vi "Math-Simple Histogram.vi"(0 "Array":dbl[](array[numeric]), 5 "Binwidth":dbl) -> (4 "Histogram Graph":T1)   [LabVIEW 2020]
uses:
  <vilib>/Analysis/NI_AALPro.lvlib
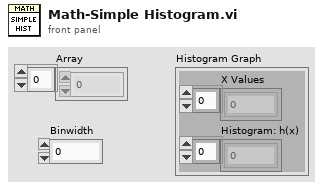
[diagram p1: front panel]
types:
  T1 = cluster{"X Values":dbl[], "Histogram: h(x)":i32[]}
  T2 = cluster{dbl, dbl, "inclusion":enum32{"lower", "upper", "both", "neither"}}
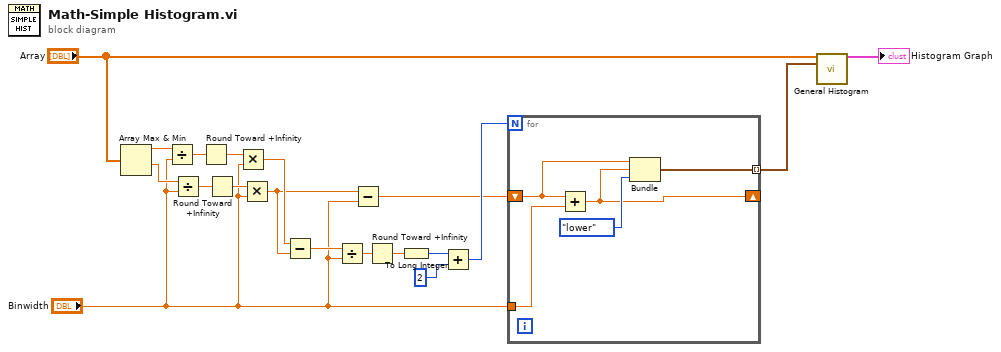
[diagram p0: block diagram]
diagram:
  n1 = Array Max & Min(array="Array") -> (max value=w9:dbl, min value=w15:dbl)  [unwired: 2 out]
  n2 = Divide(x=w9, y="Binwidth") -> (x/y=w10:dbl)
  n3 = Divide(x=w15, y="Binwidth") -> (x/y=w13:dbl)
  n4 = Round Toward +Infinity(x=w10) -> (ceil(x): smallest int >= x=w11:dbl)
  n5 = Round Toward +Infinity(x=w13) -> (ceil(x): smallest int >= x=w14:dbl)
  n6 = Multiply(x=w11, y="Binwidth") -> (x*y=w16:dbl)
  n7 = Multiply(x=w14, y="Binwidth") -> (x*y=w4:dbl)
  n8 = Subtract(x=w16, y=w4) -> (x-y=w17:dbl)
  n9 = Divide(x=w17, y="Binwidth") -> (x/y=w18:dbl)
  n10 = Subtract(x=w4, y="Binwidth") -> (x-y=w3:dbl)
  n11 = Round Toward +Infinity(x=w18) -> (ceil(x): smallest int >= x=w19:dbl)
  n12 = To Long Integer(number=w19) -> (32bit integer=w7:i32)
  n13 = Add(x=w7, y=2) -> (x+y=w5:i32)
  n14 = for {
    N: w5 -> [_]
    shift-right: [w21] -> _
    shift-left: w3 -> [w23]
    tunnel: "Binwidth" -> [w24]
    tunnel: [w20] -> w1 mode=indexing
    n15 = Add(x=w23, y=w24) -> (x+y=w21:dbl)
    n16 = Bundle(w23, w21, "inclusion"=enum32{"lower", "upper", "both", "neither"}."lower") -> (w20:T2)  [unwired: 1 in]
  }
  n17 = call <vilib>:"General Histogram.vi"("X"="Array", "Bins"=w1) -> ("Histogram Graph"=→"Histogram Graph":T1)  [unwired: 9 in, 4 out]
